vi "修改控件.vi"(8 "error in (no error)":errorcluster caption="错误输入（无错误）", 11 "程序 输入":refnum<class "程序.lvclass">) -> (0 "error out":errorcluster caption="错误输出", 3 "程序 输出":refnum<class "程序.lvclass">)   [LabVIEW 2020, in "程序.lvclass"]
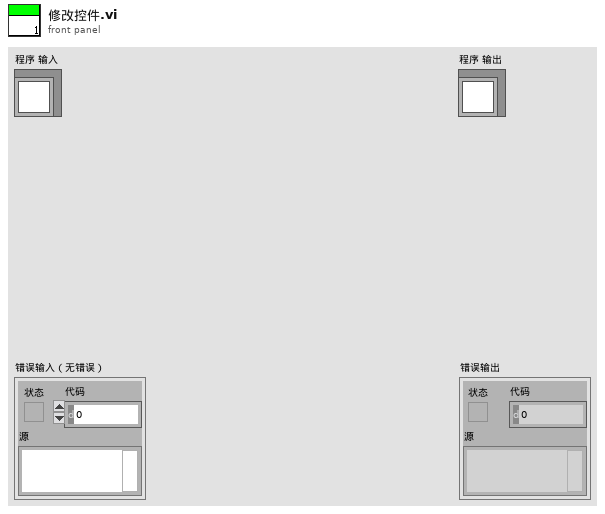
[diagram p1: front panel]
types:
  T1 = typedef "imagedata.ctl" = cluster{"image type":i32, "image depth":i32, "image":u8[], "mask":u8[], "colors":u32[], "Rectangle":cluster{"left":i16, "top":i16, "right":i16, "bottom":i16}}
  T2 = cluster{"图片":picture, "名称":string, "文本程序":string, "关键字":string, "image data":T1}[][]
  T3 = cluster{"图片":picture, "名称":string, "文本程序":string, "关键字":string, "image data":T1}
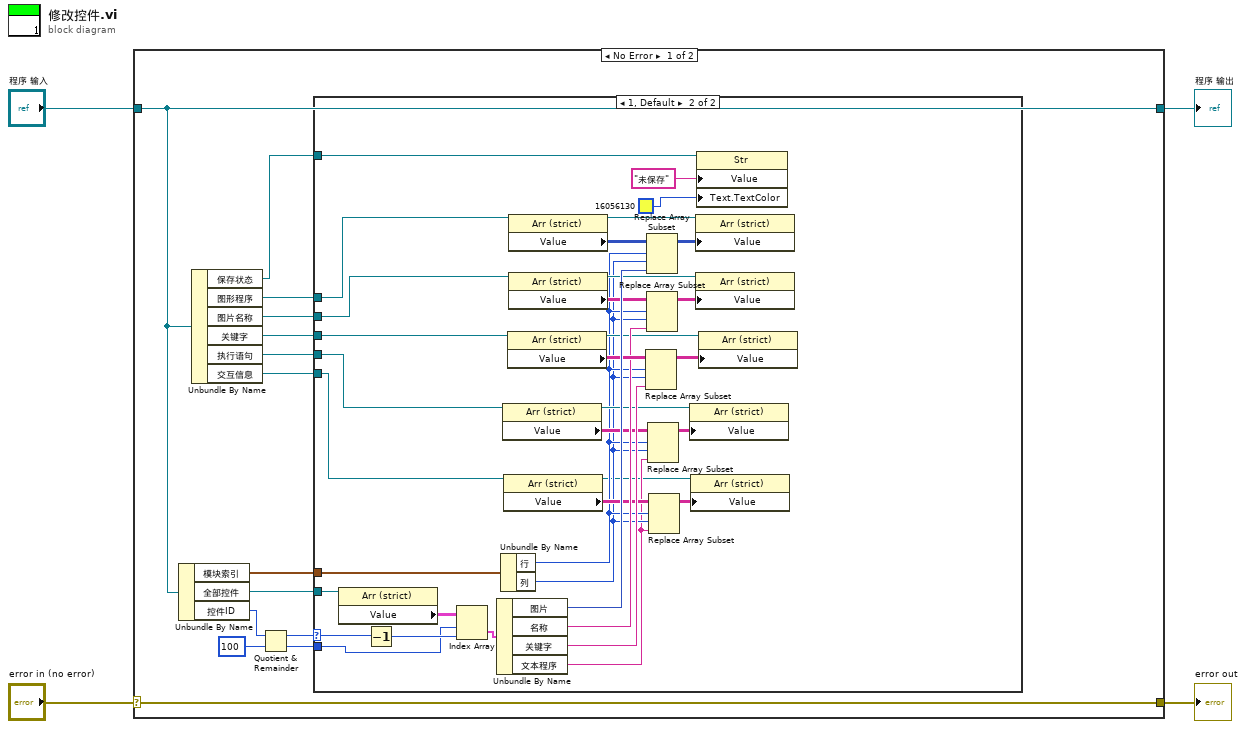
[diagram p0: block diagram]
diagram:
  n1 = case shown="No Error" "error in (no error)" {
    selector: "error in (no error)" -> [w18 w56]
    tunnel: [w18 w56] -> w3
    tunnel: [w14 w55] -> w1
    tunnel: "程序 输入" -> [w14 w55]
    frame No Error {
      n2 = Unbundle By Name(w14) -> ("模块索引"=w15:cluster{"列":u32, "行":u32}, "全部控件"=w9:refnum<vi>, "控件ID"=w17:u32)
      n3 = Unbundle By Name(w14) -> ("保存状态"=w6:refnum<vi>, "图形程序"=w13:refnum<vi>, "图片名称"=w12:refnum<vi>, "关键字"=w11:refnum<vi>, "执行语句"=w10:refnum<vi>, "交互信息"=w7:refnum<vi>)
      n4 = Quotient & Remainder(x=w17, y=u32 100) -> (x-y*floor(x/y)=w5:u32, floor(x/y)=w8:u32)
      n5 = case shown="1, Default" w5 {
        selector: w5 -> [_ w31]
        tunnel: w9 -> [_ w54]
        tunnel: w15 -> [_ w50]
        tunnel: w13 -> [_ w45]
        tunnel: w12 -> [_ w44]
        tunnel: w11 -> [_ w43]
        tunnel: w10 -> [_ w35]
        tunnel: w8 -> [_ w29]
        tunnel: w7 -> [_ w22]
        tunnel: w6 -> [_ w21]
        frame 0 {
        }
        frame 1, Default {
          n6 = property class="Arr (strict)"(reference=w54) -> ("Value"=w53:T2)  [unwired: 1 in, 2 out]
          n7 = Decrement(x=w31) -> (x-1=w30:u32)
          n8 = Index Array(array=w53, index (row)=w29, index (col)=w30) -> (element=w52:T3)
          n9 = Unbundle By Name(w52) -> ("图片"=w49:picture, "名称"=w40:string, "关键字"=w41:string, "文本程序"=w24:string)
          n10 = Unbundle By Name(w50) -> ("行"=w26:u32, "列"=w25:u32)
          n11 = property class="Arr (strict)"(reference=w35) -> (reference out=w34:refnum<vi>, "Value"=w32:string[][])  [unwired: 1 in, 1 out]
          n12 = property class="Arr (strict)"(reference=w22) -> (reference out=w23:refnum<vi>, "Value"=w27:string[][])  [unwired: 1 in, 1 out]
          n13 = property class="Arr (strict)"(reference=w43) -> (reference out=w36:refnum<vi>, "Value"=w42:string[][])  [unwired: 1 in, 1 out]
          n14 = property class="Arr (strict)"(reference=w45) -> (reference out=w48:refnum<vi>, "Value"=w51:picture[][])  [unwired: 1 in, 1 out]
          n15 = property class="Arr (strict)"(reference=w44) -> (reference out=w39:refnum<vi>, "Value"=w46:string[][])  [unwired: 1 in, 1 out]
          n16 = Replace Array Subset(array=w42, new element=w41, index (row)=w26, index (col)=w25) -> (w37:string[][])
          n17 = Replace Array Subset(array=w51, new element=w49, index (row)=w26, index (col)=w25) -> (w47:picture[][])
          n18 = Replace Array Subset(array=w46, new element=w40, index (row)=w26, index (col)=w25) -> (w38:string[][])
          n19 = Replace Array Subset(array=w32, new element=w24, index (row)=w26, index (col)=w25) -> (w33:string[][])
          n20 = Replace Array Subset(array=w27, new element=w24, index (row)=w26, index (col)=w25) -> (w28:string[][])
          n21 = property class="Arr (strict)"(reference=w34, "Value"=w33) -> ()  [unwired: 1 in, 2 out]
          n22 = property class="Arr (strict)"(reference=w23, "Value"=w28) -> ()  [unwired: 1 in, 2 out]
          n23 = property class="Arr (strict)"(reference=w48, "Value"=w47) -> ()  [unwired: 1 in, 2 out]
          n24 = property class="Arr (strict)"(reference=w39, "Value"=w38) -> ()  [unwired: 1 in, 2 out]
          n25 = property class="Str"(reference=w21, "Value"="未保存" ("值"), "Text.TextColor"=u32 16056130) -> ()  [unwired: 1 in, 2 out]
          n26 = property class="Arr (strict)"(reference=w36, "Value"=w37) -> ()  [unwired: 1 in, 2 out]
        }
      }
    }
    frame Error {
    }
  }
  "error out" <- w3
  "程序 输出" <- w1
